vi "Create DebugTools Project.vi"(8 "error in":errorcluster, 10 "CD Name":string, 11 "CDEW_MetaDataObj in":refnum<class "NIVS_CDEW_MetaDataObj.lvclass">) -> (0 "error out":errorcluster, 3 "CDEW_MetaDataObj out":refnum<class "NIVS_CDEW_MetaDataObj.lvclass">)   [LabVIEW 2026, in "NIVS_CDEW_MetaDataObj.lvclass"]
uses:
  NIVS_CDEW_MetaDataObj.lvclass
  Types/ProbeVIProjectToolStates.ctl
  NIVS_CDEW_MetaDataObj.lvclass/NIVS_CDEW_MetaDataObj.ctl
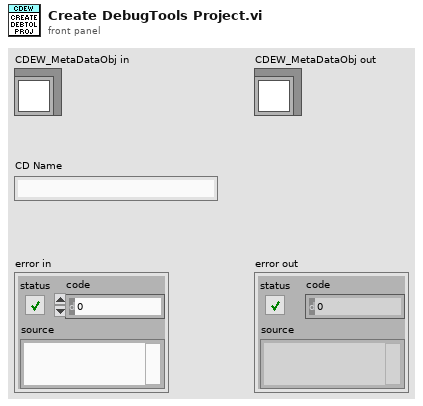
[diagram p1: front panel]
types:
  T1 = typedef "NIVS_CDEW_MetaDataObj.lvclass/ProbeVIProjectToolStates.ctl" = enum16{"CreateProbeVIsFolder", "CreateDependentFolders", "RenameProbeVIsLVLIB", "UpdateProject"}
  T2 = cluster{"DebugToolsFolderPath":path, "SourceFolderPath":path}
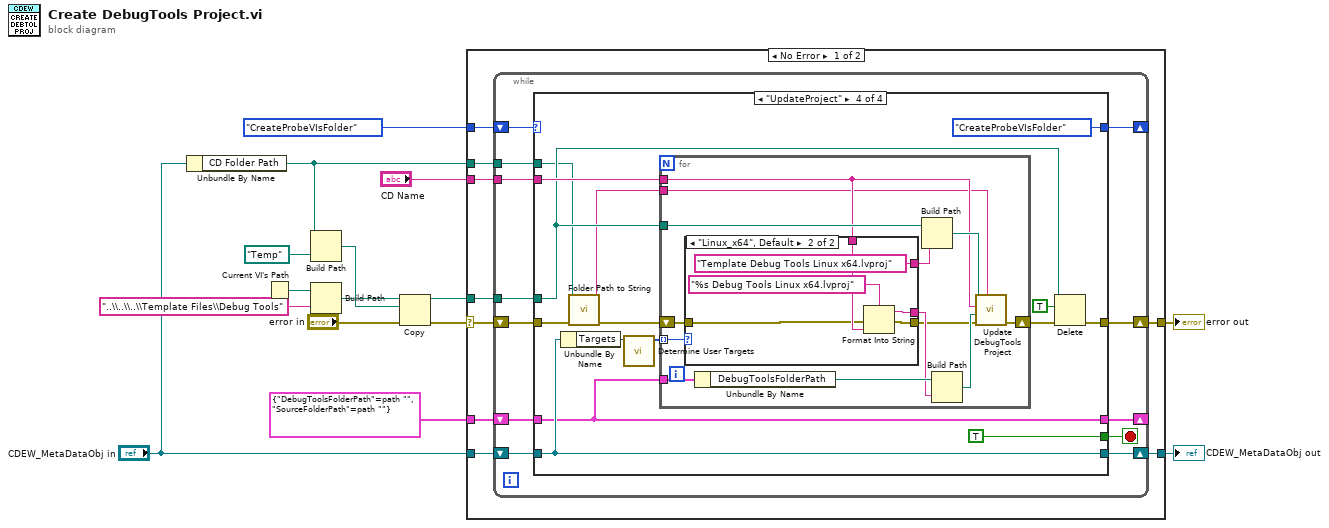
[diagram p0: block diagram]
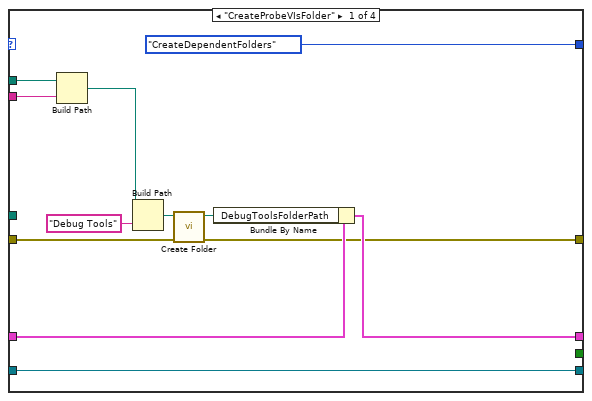
[diagram p2: hidden frame]
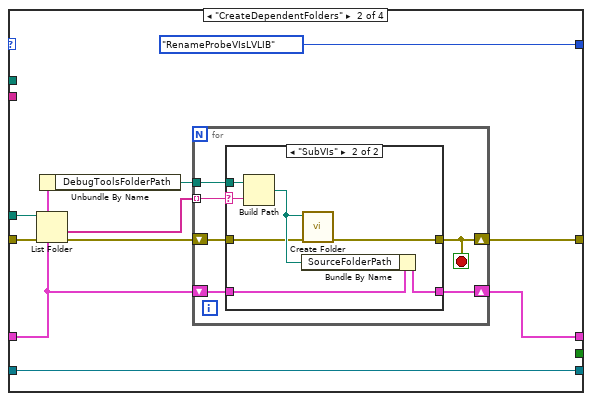
[diagram p3: hidden frame]
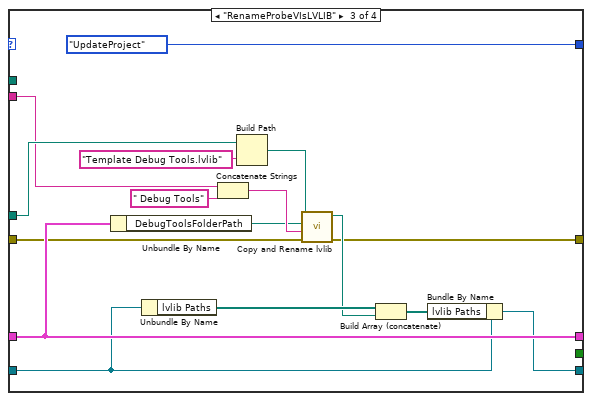
[diagram p5: hidden frame]
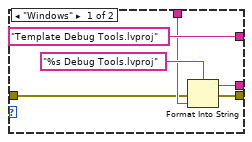
[diagram p6: hidden frame]
diagram:
  n1 = Unbundle By Name("CDEW_MetaDataObj in") -> ("CD Folder Path"=w4:path)
  n2 = Current VI's Path() -> (path=w13:path)
  n3 = Build Path(base path=w4, name or relative path=path "Temp") -> (appended path=w10:path)
  n4 = Build Path(base path=w13, name or relative path="..\\..\\..\\Template Files\\Debug Tools") -> (appended path=w9:path)
  n5 = Copy(8:"error in", 10:w10, 11:w9) -> (0:w1:errorcluster, 3:w8:path)  [unwired: 2 in, 1 out]
  n6 = case shown="No Error" w1 {
    selector: w1 -> [w16 w131]
    tunnel: T2 {"DebugToolsFolderPath"=path "", "SourceFolderPath"=path ""} -> [w24 _]
    tunnel: ProbeVIProjectToolStates."CreateProbeVIsFolder" ("Enum") -> [w23 _]
    tunnel: w8 -> [w22 _]
    tunnel: "CDEW_MetaDataObj in" -> [w21 w130]
    tunnel: [w20 w130] -> w6
    tunnel: "CD Name" -> [w19 _]
    tunnel: w4 -> [w18 _]
    tunnel: [w17 w131] -> w3
    frame No Error {
      n7 = while {
        shift-right: [w30] -> _
        shift-left: w23 -> [w36]
        tunnel: w19 -> [w35]
        shift-right: [w33] -> _
        shift-left: w24 -> [w34]
        tunnel: w22 -> [w32]
        shift-right: [w28] -> w20
        shift-left: w21 -> [w29]
        tunnel: w18 -> [w27]
        shift-right: [w26] -> w17
        shift-left: w16 -> [w25]
        stop <- w31 stop-if-true
        n8 = case shown="\"UpdateProject\"" w36 {
          tunnel: w35 -> [w38 _ w85 w103]
          tunnel: w34 -> [w48 w55 w84 w96]
          tunnel: [w47 w56 w84 w96] -> w33
          tunnel: w32 -> [_ w58 w89 w101]
          tunnel: [ProbeVIProjectToolStates."CreateDependentFolders" ("Enum") ProbeVIProjectToolStates."RenameProbeVIsLVLIB" ("Enum") ProbeVIProjectToolStates."UpdateProject" ("Enum") ProbeVIProjectToolStates."CreateProbeVIsFolder" ("Enum")] -> w30
          tunnel: [_ _ _ TRUE] -> w31
          tunnel: w29 -> [w43 w52 w76 w99]
          tunnel: [w43 w52 w77 w99] -> w28
          tunnel: w27 -> [w39 _ _ w95]
          tunnel: [w41 w49 w74 w90] -> w26
          tunnel: w25 -> [w40 w51 w75 w94]
          frame "CreateProbeVIsFolder" {
            n9 = Build Path(base path=w39, name or relative path=w38) -> (appended path=w37:path)
            n10 = Build Path(base path=w37, name or relative path="Debug Tools" ("string")) -> (appended path=w45:path)
            n11 = call "Create Folder.vi"("error in"=w40, "Folder Path"=w45) -> ("error out"=w41:errorcluster, "Folder Path Out"=w46:path)  [unwired: 8 in]
            n12 = Bundle By Name(cluster=w48, "DebugToolsFolderPath"=w46) -> (w47:T2)
          }
          frame "CreateDependentFolders" {
            n13 = List Folder(path=w58, error in=w51) -> (folder names=w57:string[], error out=w50:errorcluster)  [unwired: 2 in, 2 out]
            n14 = Unbundle By Name(w55) -> ("DebugToolsFolderPath"=w54:path)
            n15 = for {
              tunnel: w57 -> [w64] mode=indexing
              shift-right: [w62] -> w56
              shift-left: w55 -> [w63]
              tunnel: w54 -> [w61]
              shift-right: [w59] -> w49
              shift-left: w50 -> [w60]
              stop <- w59 stop-if-true
              n16 = case shown="\"SubVIs\"" w64 {
                selector: w64 -> [_ w69]
                tunnel: w61 -> [_ w73]
                tunnel: w63 -> [w66 w72]
                tunnel: [w66 w71] -> w62
                tunnel: w60 -> [w65 w68]
                tunnel: [w65 w67] -> w59
                frame Default {
                }
                frame "SubVIs" {
                  n17 = Build Path(base path=w73, name or relative path=w69) -> (appended path=w70:path)
                  n18 = Bundle By Name(cluster=w72, "SourceFolderPath"=w70) -> (w71:T2)
                  n19 = call "Create Folder.vi"("error in"=w68, "Folder Path"=w70) -> ("error out"=w67:errorcluster)  [unwired: 8 in, 1 out]
                }
              }
            }
          }
          frame "RenameProbeVIsLVLIB" {
            n20 = Unbundle By Name(w84) -> ("DebugToolsFolderPath"=w81:path)
            n21 = Unbundle By Name(w76) -> ("lvlib Paths"=w80:path[])
            n22 = Concatenate Strings(w85, " Debug Tools" ("string")) -> (w82:string)
            n23 = Build Path(base path=w89, name or relative path="Template Debug Tools.lvlib" ("string")) -> (appended path=w87:path)
            n24 = call "Copy and Rename lvlib.vi"("error in"=w75, "New lvlib Name"=w82, "Destination Directory Path"=w81, "lvlib Path"=w87) -> ("error out"=w74:errorcluster, "New Library Path"=w79:path)  [unwired: 6 in]
            n25 = Build Array (concatenate)(w80, w79) -> (w78:path[])
            n26 = Bundle By Name(cluster=w76, "lvlib Paths"=w78) -> (w77:refnum<class "NIVS_CDEW_MetaDataObj.lvclass">)
          }
          frame "UpdateProject" {
            n27 = Unbundle By Name(w99) -> ("Targets"=w98:enum16{"Linux_x64", "Windows", "Both"})
            n28 = call "Folder Path to String.vi"("error in"=w94, "CD Folder Path"=w95) -> ("error out"=w93:errorcluster, "Path as String"=w92:string)  [unwired: 8 in]
            n29 = call "Determine User Targets.vi"("Targets"=w98) -> ("User Configured Targets"=w97:enum16{"Linux_x64", "Windows", "Both"}[])  [unwired: 10 in]
            n30 = for {
              tunnel: w103 -> [w113]
              tunnel: w101 -> [w116]
              tunnel: w97 -> [w115] mode=indexing
              tunnel: w96 -> [w112]
              shift-right: [w106] -> w91
              shift-left: w93 -> [w108]
              tunnel: w92 -> [w105]
              n31 = case shown="\"Linux_x64\", Default" w115 {
                tunnel: ["Template Debug Tools.lvproj" ("Custom Device Name") "Template Debug Tools Linux x64.lvproj" ("Custom Device Name")] -> w114
                tunnel: w113 -> [w121 w127]
                tunnel: [w120 w126] -> w110
                tunnel: w108 -> [w119 w125]
                tunnel: [w118 w124] -> w107
                frame "Windows" {
                  n32 = Format Into String(format string="%s Debug Tools.lvproj", error in=w119, w121) -> (resulting string=w120:string, error out=w118:errorcluster)  [unwired: 1 in]
                }
                frame "Linux_x64", Default {
                  n33 = Format Into String(format string="%s Debug Tools Linux x64.lvproj", error in=w125, w127) -> (resulting string=w126:string, error out=w124:errorcluster)  [unwired: 1 in]
                }
              }
              n34 = Unbundle By Name(w112) -> ("DebugToolsFolderPath"=w111:path)
              n35 = Build Path(base path=w116, name or relative path=w114) -> (appended path=w117:path)
              n36 = Build Path(base path=w111, name or relative path=w110) -> (appended path=w109:path)
              n37 = call "Update DebugTools Project.vi"("CD Folder Path"=w105, "error in"=w107, "DebugTools Project Path"=w109, "CD Name"=w113, "Project path"=w117) -> ("error out"=w106:errorcluster)  [unwired: 6 in]
            }
            n38 = Delete(path (use dialog)=w101, entire hierarchy (F)=TRUE, error in=w91) -> (error out=w90:errorcluster)  [unwired: 2 in, 2 out]
          }
        }
      }
    }
    frame Error {
    }
  }
  "CDEW_MetaDataObj out" <- w6
  "error out" <- w3
